vi "Nominal Value Write Array.vi"(0 "Power Nominal Value in":refnum<class "Power Nominal Value.lvclass">, 1 "Power Nominal Value Value":dbl[](array[numeric]), 3 "error in":errorcluster) -> (7 "Power Nominal Value out":refnum<class "Power Nominal Value.lvclass">, 10 "error out":errorcluster)   [LabVIEW 2023, in "Power Nominal Value.lvclass"]
uses:
  Power Nominal Value.lvclass
  Power Nominal Value.lvclass/Power Nominal Value.ctl
  Parents/Nominal Value/Nominal Value.lvclass
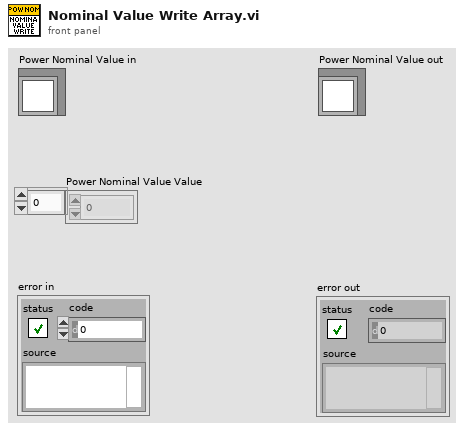
[diagram p1: front panel]
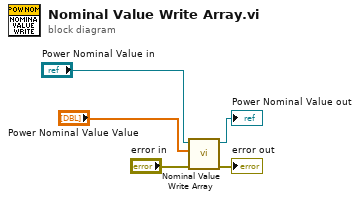
[diagram p0: block diagram]
diagram:
  n1 = call-parent "Nominal Value Write Array.vi"("Nominal Value in"="Power Nominal Value in", "Nominal Value Value"="Power Nominal Value Value", "error in"="error in") -> ("Nominal Value out"=→"Power Nominal Value out":refnum<class "Power Nominal Value.lvclass">, "error out"=→"error out":errorcluster)  [unwired: 6 in]
